vi "flat_secuence.vi"() -> ()   [LabVIEW 2020]
panel:
  out "Tank 4":u8(slide) scale=0.0..100.0
  out "Tank 3":u8(slide) scale=0.0..100.0
  out "Tank 2":u8(slide) scale=0.0..100.0
  out "Tank 1":u8(slide) scale=0.0..100.0
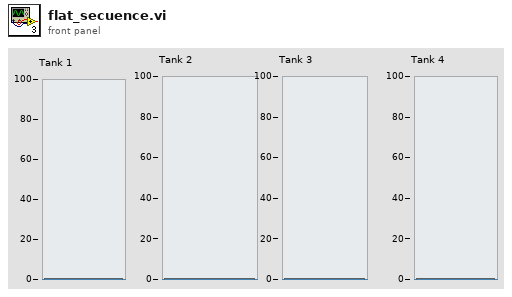
[diagram p1: front panel]
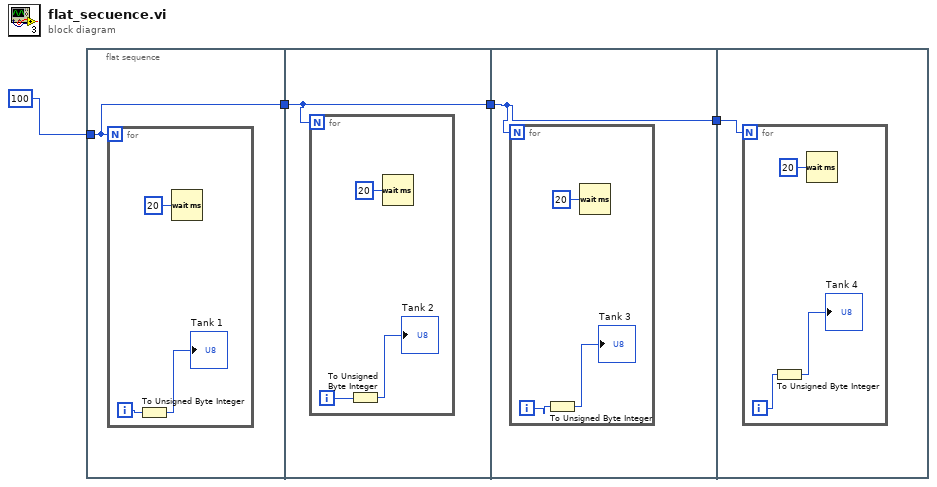
[diagram p0: block diagram]
diagram:
  n1 = flat-sequence {
    tunnel: 100 -> [w5]
    tunnel: [w5] -> w3
    tunnel: w3 -> [w9]
    tunnel: [w9] -> w2
    tunnel: w2 -> [w13]
    tunnel: [w13] -> w1
    tunnel: w1 -> [w17]
    frame #0 {
      n2 = for {
        N: w5 -> [_]
        i -> [w8]
        n3 = To Unsigned Byte Integer(number=w8) -> (unsigned 8bit integer=→"Tank 1":u8)
        n4 = Wait (ms)(milliseconds to wait=u32 20) -> ()  [unwired: 1 out]
      }
    }
    frame #1 {
      n5 = for {
        N: w9 -> [_]
        i -> [w10]
        n6 = To Unsigned Byte Integer(number=w10) -> (unsigned 8bit integer=→"Tank 2":u8)
        n7 = Wait (ms)(milliseconds to wait=u32 20) -> ()  [unwired: 1 out]
      }
    }
    frame #2 {
      n8 = for {
        N: w13 -> [_]
        i -> [w14]
        n9 = To Unsigned Byte Integer(number=w14) -> (unsigned 8bit integer=→"Tank 3":u8)
        n10 = Wait (ms)(milliseconds to wait=u32 20) -> ()  [unwired: 1 out]
      }
    }
    frame #3 {
      n11 = for {
        N: w17 -> [_]
        i -> [w18]
        n12 = To Unsigned Byte Integer(number=w18) -> (unsigned 8bit integer=→"Tank 4":u8)
        n13 = Wait (ms)(milliseconds to wait=u32 20) -> ()  [unwired: 1 out]
      }
    }
  }
